vi "PI.vi"(4 "Tasking Period":dbl, 5 "Kp":dbl, 6 "Reference Speed (rad/s)":dbl, 7 "Ki":dbl, 8 "Real Speed (rad/s)":dbl, 11 "Error In":errorcluster) -> (1 "PI Current (A)":dbl, 3 "Error Out":errorcluster)   [LabVIEW 2021]
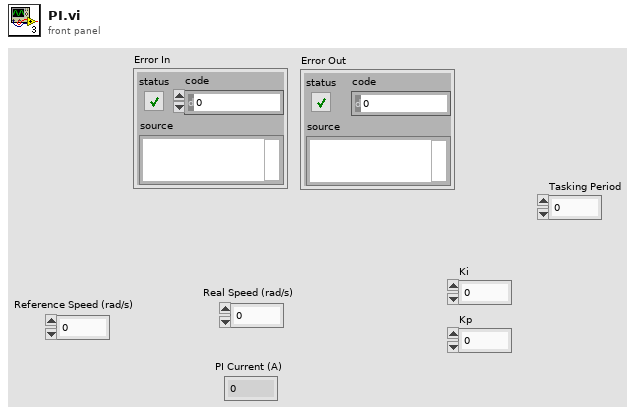
[diagram p1: front panel]
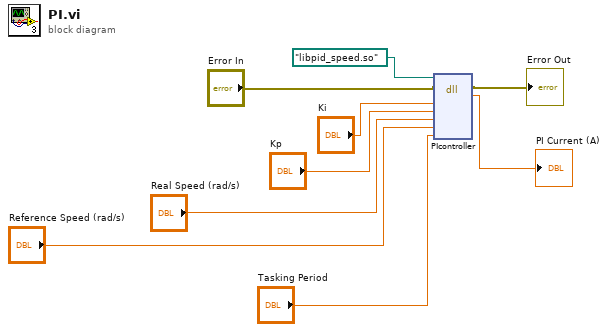
[diagram p0: block diagram]
diagram:
  n1 = dll-call lib="?" fn="PIcontroller"(path in=path "libpid_speed.so", error in="Error In", "Ki"="Ki", "Kp"="Kp", "measured_speed"="Real Speed (rad/s)", "reference_speed"="Reference Speed (rad/s)", "Tasking_period"="Tasking Period") -> (error out=→"Error Out":errorcluster, "output"=→"PI Current (A)":sgl)  [unwired: 6 in, 1 out]
